vi "DBM Reference.vi"() -> ()   [LabVIEW 2020]
panel:
  in  "탭 컨트롤":enum32{"수심 - 압력 변환", "페이지 2"}(tab)
  in  "변환2":bool
  in  "변환1":bool
  in  "수심 (m)":dbl
  in  "압력 (kPa)":dbl
  # "* 물온도 15 ℃ 기준"
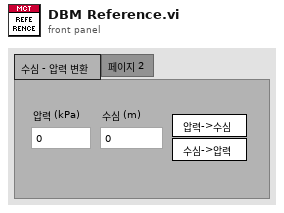
[diagram p1: front panel]
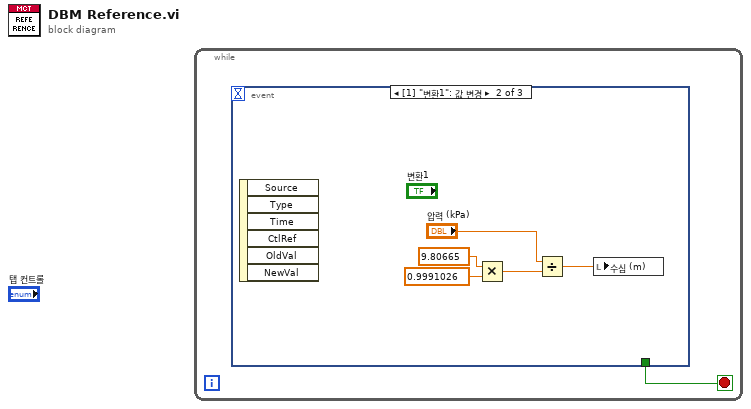
[diagram p0: block diagram]
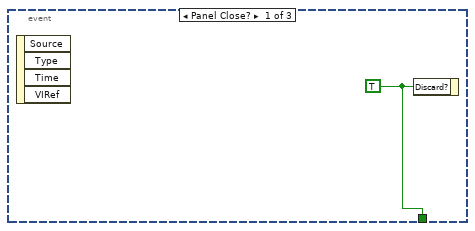
[diagram p2: hidden frame]
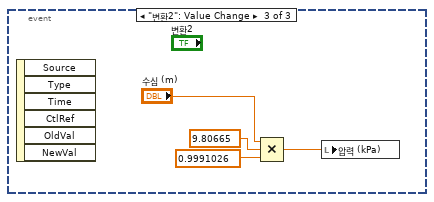
[diagram p3: hidden frame]
diagram:
  n1 = while {
    stop <- w1 stop-if-true
    n2 = event shown="[1] \"변환1\": 값 변경" {
      selector: _ -> [_ _ _]
      dyn-events: _ -> [_ _ _]
      timeout: _ -> [_ _ _]
      tunnel: [w2 _ _] -> w1
      event Panel Close? {
        w2 = TRUE ("버림?")
        n3 = event-data() -> ()  [unwired: 1 in, 4 out]
        n4 = event-data("Discard?"=w2) -> ()  [unwired: 1 in, 1 out]
      }
      event "변환1": Value Change {
        n5 = event-data() -> ()  [unwired: 1 in, 6 out]
        n6 = Multiply(x=9.80665, y=0.9991026) -> (x*y=w5:dbl)
        n7 = Divide(x="압력 (kPa)", y=w5) -> (x/y=w3:dbl)
        n8 = local write "수심 (m)"(w3) -> ()
      }
      event "변환2": Value Change {
        n9 = event-data() -> ()  [unwired: 1 in, 6 out]
        n10 = Compound Arithmetic op=MULTIPLY("수심 (m)", 9.80665 ("x"), 0.9991026 ("y")) -> (w8:dbl)
        n11 = local write "압력 (kPa)"(w8) -> ()
      }
    }
  }
